vi "DriverStationGetCommands.vi"() -> ()   [LabVIEW 2020]
doc: "This VI receives instructions from the driver and manipulator controls, but only in certain robot modes. Specifically, these instructions are received while the robot is either \"running autonomously\" or in Super Test Mode. In all other robot modes, no instructions are received via the driver station. Instead they are output by the Autonomous Sequencer or completely disabled."
uses:
  refnumbers.vi
  GRNF_Joystick.vi
  driverdata.vi
  <vilib>/Rock Robotics/Network Tables/NT Read Boolean Array.vi
  <vilib>/Rock Robotics/Network Tables/NT Read Boolean.vi
  drivercommands.vi
panel:
  in  "Buttons":bool[](array[boolean])=[FALSE, FALSE, FALSE, FALSE, FALSE, FALSE, FALSE, FALSE, FALSE, FALSE]
  in  "Right Trigger":dbl(slide) min=0.0 max=1.0 scale=0.0..1.0
  in  "Left Trigger":dbl(slide) min=0.0 max=1.0 step=0.1 scale=0.0..1.0
  in  "Right Joystick X":dbl(slide) scale=-1.0..1.0
  in  "Enable Joystick Control Override":bool
  in  "Joystick Left X":dbl(slide) scale=-1.0..1.0
  in  "Joystick Left Y":dbl(slide) scale=1.0..-1.0
  in  "Joystick Right Y":dbl(slide) scale=1.0..-1.0
  # "Left Thumbstick"
  # "Right Thumbstick"
  # "Driver A"
  # "Driver B"
  # "Driver X"
  # "Driver Y"
  # "Driver Left Bumper"
  # "Driver Right Bumper"
  # "Driver View"
  # "Driver Menu"
  # "Driver Left Joystick Button"
  # "Driver Right Joystick Button"
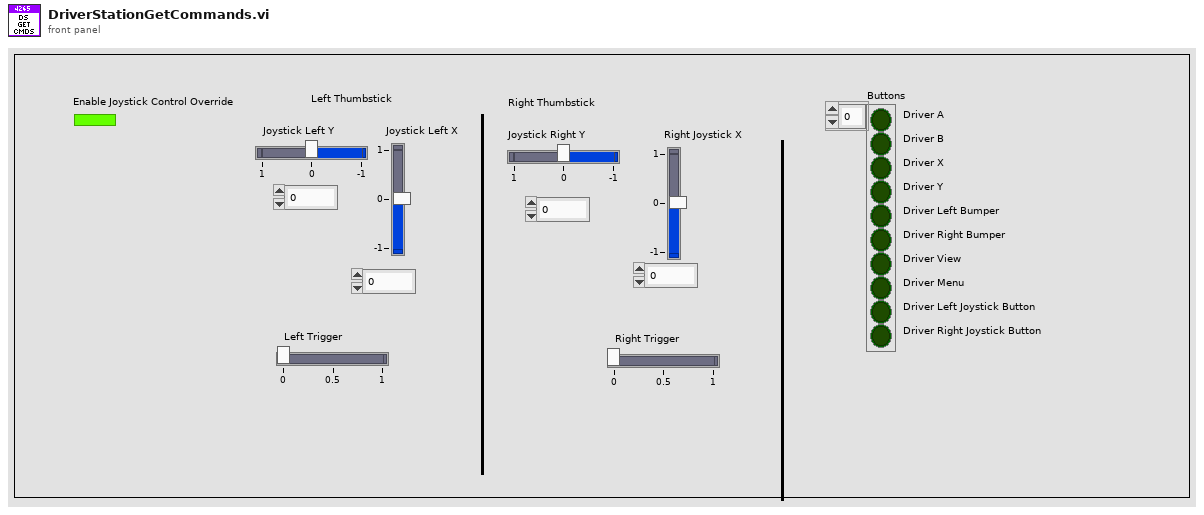
[diagram p1: front panel]
types:
  T1 = typedef "WPI_JoystickDevRef.ctl" = cluster{"Device":T2}
  T2 = typedef "WPI_JoystickDeviceEnum.ctl" = enum16{"USB 0", "USB 1", "USB 2", "USB 3", "USB 4", "USB 5"}
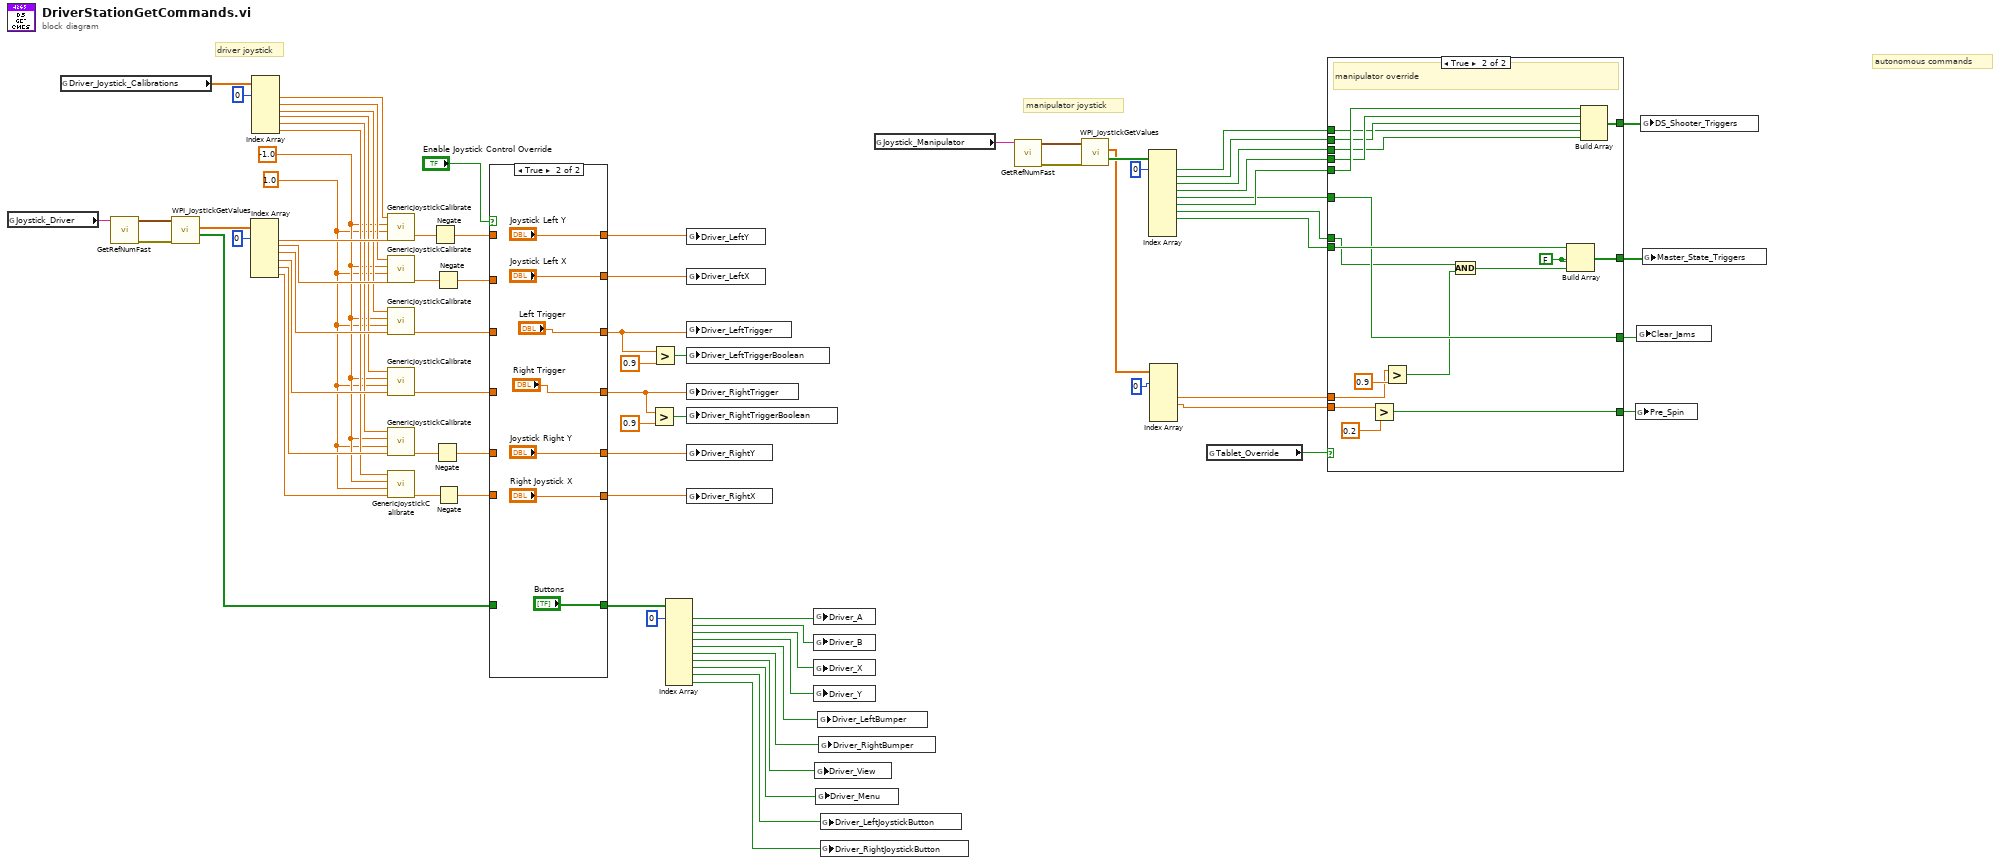
[diagram p0: block diagram]
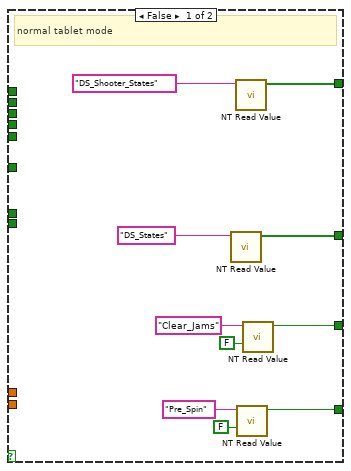
[diagram p3: hidden frame]
diagram:
  w36 = 1.0
  w37 = -1.0
  # "autonomous commands"
  # "manipulator joystick"
  # "driver joystick"
  n1 = global read "refnumbers.vi" "Joystick_Driver"() -> (w60:string)
  n2 = global read "driverdata.vi" "Driver_Joystick_Calibrations"() -> (w54:dbl[])
  n3 = call-poly "GetRefNumFast.vi"("RefNum Name"=w60) -> ("Error"=w61:errorcluster, "Device Reference"=w62:T1)  [unwired: 5 in]
  n4 = call <vilib>:"WPI_JoystickGetValues.vi"("error in (no error)"=w61, "JoystickDevRef"=w62) -> ("Buttons"=w18:bool[], "Axes"=w77:dbl[])  [unwired: 5 in, 3 out]
  n5 = Index Array(array=w77, index #1=0 ("index")) -> (element #1=w49:dbl, element #2=w48:dbl, element #3=w44:dbl, element #4=w45:dbl, element #5=w46:dbl, element #6=w47:dbl)  [unwired: 5 in]
  n6 = Index Array(array=w54, index #1=0 ("index")) -> (element #1=w38:dbl, element #2=w39:dbl, element #3=w40:dbl, element #4=w41:dbl, element #5=w42:dbl, element #6=w43:dbl)  [unwired: 5 in]
  n7 = call "GenericJoystickCalibrate.vi"("Raw Joystick Value"=w49, "Maximum"=w36, "Minimum"=w37, "Deadband"=w38) -> ("Scaled Joystick Value"=w53:dbl)  [unwired: 3 in]
  n8 = call "GenericJoystickCalibrate.vi"("Raw Joystick Value"=w48, "Maximum"=w36, "Minimum"=w37, "Deadband"=w39) -> ("Scaled Joystick Value"=w52:dbl)  [unwired: 3 in]
  n9 = call "GenericJoystickCalibrate.vi"("Raw Joystick Value"=w44, "Maximum"=w36, "Minimum"=w37, "Deadband"=w40) -> ("Scaled Joystick Value"=w30:dbl)  [unwired: 3 in]
  n10 = call "GenericJoystickCalibrate.vi"("Raw Joystick Value"=w45, "Maximum"=w36, "Minimum"=w37, "Deadband"=w41) -> ("Scaled Joystick Value"=w24:dbl)  [unwired: 3 in]
  n11 = call "GenericJoystickCalibrate.vi"("Raw Joystick Value"=w46, "Maximum"=w36, "Minimum"=w37, "Deadband"=w42) -> ("Scaled Joystick Value"=w51:dbl)  [unwired: 3 in]
  n12 = call "GenericJoystickCalibrate.vi"("Raw Joystick Value"=w47, "Maximum"=w36, "Minimum"=w37, "Deadband"=w43) -> ("Scaled Joystick Value"=w50:dbl)  [unwired: 3 in]
  n13 = Negate(x=w53) -> (-x=w33:dbl)
  n14 = Negate(x=w51) -> (-x=w21:dbl)
  n15 = Negate(x=w52) -> (-x=w32:dbl)
  n16 = Negate(x=w50) -> (-x=w20:dbl)
  n17 = case shown="True" "Enable Joystick Control Override" {
    tunnel: w30 -> [w82 _]
    tunnel: [w84 "Joystick Left Y"] -> w34
    tunnel: w33 -> [w84 _]
    tunnel: [w83 "Joystick Left X"] -> w31
    tunnel: w32 -> [w83 _]
    tunnel: [w82 "Left Trigger"] -> w25
    tunnel: w24 -> [w81 _]
    tunnel: [w81 "Right Trigger"] -> w23
    tunnel: [w80 "Joystick Right Y"] -> w22
    tunnel: w21 -> [w80 _]
    tunnel: [w79 "Right Joystick X"] -> w19
    tunnel: w20 -> [w79 _]
    tunnel: w18 -> [w78 _]
    tunnel: [w78 "Buttons"] -> w17
    frame False {
    }
    frame True {
    }
  }
  n18 = Greater?(x=w23, y=0.9) -> (0:w27:bool)
  n19 = Greater?(x=w25, y=0.9) -> (0:w26:bool)
  n20 = Index Array(array=w17, index #1=0 ("index")) -> (element #1=w74:bool, element #2=w73:bool, element #3=w72:bool, element #4=w71:bool, element #5=w70:bool, element #6=w69:bool, element #7=w68:bool, element #8=w67:bool, element #9=w66:bool, element #10=w65:bool)  [unwired: 9 in]
  n21 = global write "drivercommands.vi" "Driver_LeftY"(w34) -> ()
  n22 = global write "drivercommands.vi" "Driver_LeftX"(w31) -> ()
  n23 = global write "drivercommands.vi" "Driver_LeftTrigger"(w25) -> ()
  n24 = global write "drivercommands.vi" "Driver_LeftTriggerBoolean"(w26) -> ()
  n25 = global write "drivercommands.vi" "Driver_RightTrigger"(w23) -> ()
  n26 = global write "drivercommands.vi" "Driver_RightTriggerBoolean"(w27) -> ()
  n27 = global write "drivercommands.vi" "Driver_RightY"(w22) -> ()
  n28 = global write "drivercommands.vi" "Driver_RightX"(w19) -> ()
  n29 = global write "drivercommands.vi" "Driver_A"(w74) -> ()
  n30 = global write "drivercommands.vi" "Driver_B"(w73) -> ()
  n31 = global write "drivercommands.vi" "Driver_X"(w72) -> ()
  n32 = global write "drivercommands.vi" "Driver_Y"(w71) -> ()
  n33 = global write "drivercommands.vi" "Driver_View"(w68) -> ()
  n34 = global write "drivercommands.vi" "Driver_Menu"(w67) -> ()
  n35 = global write "drivercommands.vi" "Driver_LeftBumper"(w70) -> ()
  n36 = global write "drivercommands.vi" "Driver_RightBumper"(w69) -> ()
  n37 = global write "drivercommands.vi" "Driver_LeftJoystickButton"(w66) -> ()
  n38 = global write "drivercommands.vi" "Driver_RightJoystickButton"(w65) -> ()
  n39 = global read "refnumbers.vi" "Joystick_Manipulator"() -> (w57:string)
  n40 = call-poly "GetRefNumFast.vi"("RefNum Name"=w57) -> ("Error"=w58:errorcluster, "Device Reference"=w59:T1)  [unwired: 5 in]
  n41 = call <vilib>:"WPI_JoystickGetValues.vi"("error in (no error)"=w58, "JoystickDevRef"=w59) -> ("Buttons"=w13:bool[], "Axes"=w3:dbl[])  [unwired: 5 in, 3 out]
  n42 = Index Array(array=w13, index #1=0 ("index")) -> (element #1=w7:bool, element #2=w8:bool, element #3=w6:bool, element #4=w9:bool, element #5=w5:bool, element #6=w10:bool, element #7=w11:bool, element #8=w12:bool)  [unwired: 9 in, 2 out]
  n43 = Index Array(array=w3, index #1=0 ("index")) -> (element #3=w1:dbl, element #4=w2:dbl)  [unwired: 5 in, 4 out]
  n44 = global read "driverdata.vi" "Tablet_Override"() -> (w63:bool)
  n45 = case shown="True" w63 {
    tunnel: [w100 w119] -> w64
    tunnel: [w97 w110] -> w56
    tunnel: [w94 w107] -> w16
    tunnel: [w92 w116] -> w15
    tunnel: w12 -> [_ w117]
    tunnel: w11 -> [_ w104]
    tunnel: w10 -> [_ w115]
    tunnel: w9 -> [_ w114]
    tunnel: w8 -> [_ w113]
    tunnel: w7 -> [_ w112]
    tunnel: w6 -> [_ w111]
    tunnel: w5 -> [_ w110]
    tunnel: w2 -> [_ w108]
    tunnel: w1 -> [_ w105]
    frame False {
      # "normal tablet mode"
      n46 = call-poly <vilib>:"NT Read Value.vi"("Name"="DS_States" ("refnum name")) -> ("Boolean Array"=w100:bool[])  [unwired: 9 in, 1 out]
      n47 = call-poly <vilib>:"NT Read Value.vi"("Name"="DS_Shooter_States" ("refnum name")) -> ("Boolean Array"=w92:bool[])  [unwired: 9 in, 1 out]
      n48 = call-poly <vilib>:"NT Read Value.vi"("Default Value"=FALSE, "Name"="Pre_Spin" ("refnum name")) -> ("Boolean"=w94:bool)  [unwired: 8 in, 1 out]
      n49 = call-poly <vilib>:"NT Read Value.vi"("Default Value"=FALSE, "Name"="Clear_Jams" ("refnum name")) -> ("Boolean"=w97:bool)  [unwired: 8 in, 1 out]
    }
    frame True {
      w118 = FALSE
      # "manipulator override"
      n50 = Greater?(x=w108, y=0.2) -> (0:w107:bool)
      n51 = Greater?(x=w105, y=0.9) -> (0:w103:bool)
      n52 = And(x=w104, y=w103) -> (x .and. y?=w102:bool)
      n53 = Build Array(w117, w118, w118, w102) -> (w119:bool[])
      n54 = Build Array(w115, w114, w113, w112, w111) -> (w116:bool[])
    }
  }
  n55 = global write "drivercommands.vi" "Pre_Spin"(w16) -> ()
  n56 = global write "drivercommands.vi" "Clear_Jams"(w56) -> ()
  n57 = global write "drivercommands.vi" "DS_Shooter_Triggers"(w15) -> ()
  n58 = global write "drivercommands.vi" "Master_State_Triggers"(w64) -> ()
